vi "RDB Init New Message.vi"(7 "RDB Receive Reference.RDB Signals":dbl[](array[numeric]), 8 "error in (no error)":errorcluster, 10 "RDB Reference in":T4 {"RDB Send Reference"."RDB Data"."payload" format="%x"; "RDB Send Reference"."RDB Data"."timestamp" format="%<%.7X\n%x>T"; "RDB Send Reference"."RDB Data"."type" items=["FlexRay Data"=32, "FlexRay Null"=33, "FlexRay Symbol"=34, "Log Trigger"=225, "Start Trigger"=226]; "RDB Send Reference"."RDB Data"."cycle count" max=63 step=1; "RDB Receive Reference"."RDB Data"."payload" format="%x"; "RDB Receive Reference"."RDB Data"."timestamp" format="%<%.7X\n%x>T"; "RDB Receive Reference"."RDB Data"."type" items=["FlexRay Data"=32, "FlexRay Null"=33, "FlexRay Symbol"=34, "Log Trigger"=225, "Start Trigger"=226]; "RDB Receive Reference"."RDB Data"."cycle count" max=63 step=1}, 11 "Settings":T1={"UDP Receiver"=refnum, "UDP Sender"=refnum, "Valid Packet"=FALSE, "TCP"=refnum, "Network Settings"={"IP adress"="127.0.0.1", "RDB"={"Protocol"=enum."UDP", "Tx Port"=48270, "Rx Port"=10, "Buffer Size"=204800, "Timeout"=10}, "SCP"={"Protocol"=enum."TCP", "Tx Port"=48191, "Rx Port"=48191, "Buffer Size"=204800, "Timeout"=10}}, "vclient"=path ""}) -> (0 "error out":errorcluster, 2 "RDB Reference out":T4 {"RDB Send Reference"."RDB Data"."payload" format="%x"; "RDB Send Reference"."RDB Data"."timestamp" format="%<%.7X\n%x>T"; "RDB Send Reference"."RDB Data"."type" items=["FlexRay Data"=32, "FlexRay Null"=33, "FlexRay Symbol"=34, "Log Trigger"=225, "Start Trigger"=226]; "RDB Send Reference"."RDB Data"."cycle count" max=63 step=1; "RDB Receive Reference"."RDB Data"."payload" format="%x"; "RDB Receive Reference"."RDB Data"."timestamp" format="%<%.7X\n%x>T"; "RDB Receive Reference"."RDB Data"."type" items=["FlexRay Data"=32, "FlexRay Null"=33, "FlexRay Symbol"=34, "Log Trigger"=225, "Start Trigger"=226]; "RDB Receive Reference"."RDB Data"."cycle count" max=63 step=1}, 3 "Settings":T1={"UDP Receiver"=refnum, "UDP Sender"=refnum, "Valid Packet"=FALSE, "TCP"=refnum, "Network Settings"={"IP adress"="127.0.0.1", "RDB"={"Protocol"=enum."UDP", "Tx Port"=48270, "Rx Port"=10, "Buffer Size"=204800, "Timeout"=10}, "SCP"={"Protocol"=enum."TCP", "Tx Port"=48191, "Rx Port"=48191, "Buffer Size"=204800, "Timeout"=10}}, "vclient"=path ""})   [LabVIEW 2020, in "RDB.lvlib"]
uses:
  RDB.lvlib
  RDB References.ctl
  RDB Reference.ctl
  <vilib>/xnet/xnet.llb/XNET Frame FlexRay.ctl
  <vilib>/xnet/xnet.llb/XNET Frame Type FlexRay.ctl
  Engine/Type/Settings.ctl
  Shared/Network Settings.ctl
  Shared/Protocol.ctl
  <vilib>/xnet/xnet.llb/XNET Convert (Signal to Frame FlexRay).vi
  Shared/Vires VTD Shared.lvlib
  Engine/Vires VTD Engine.lvlib
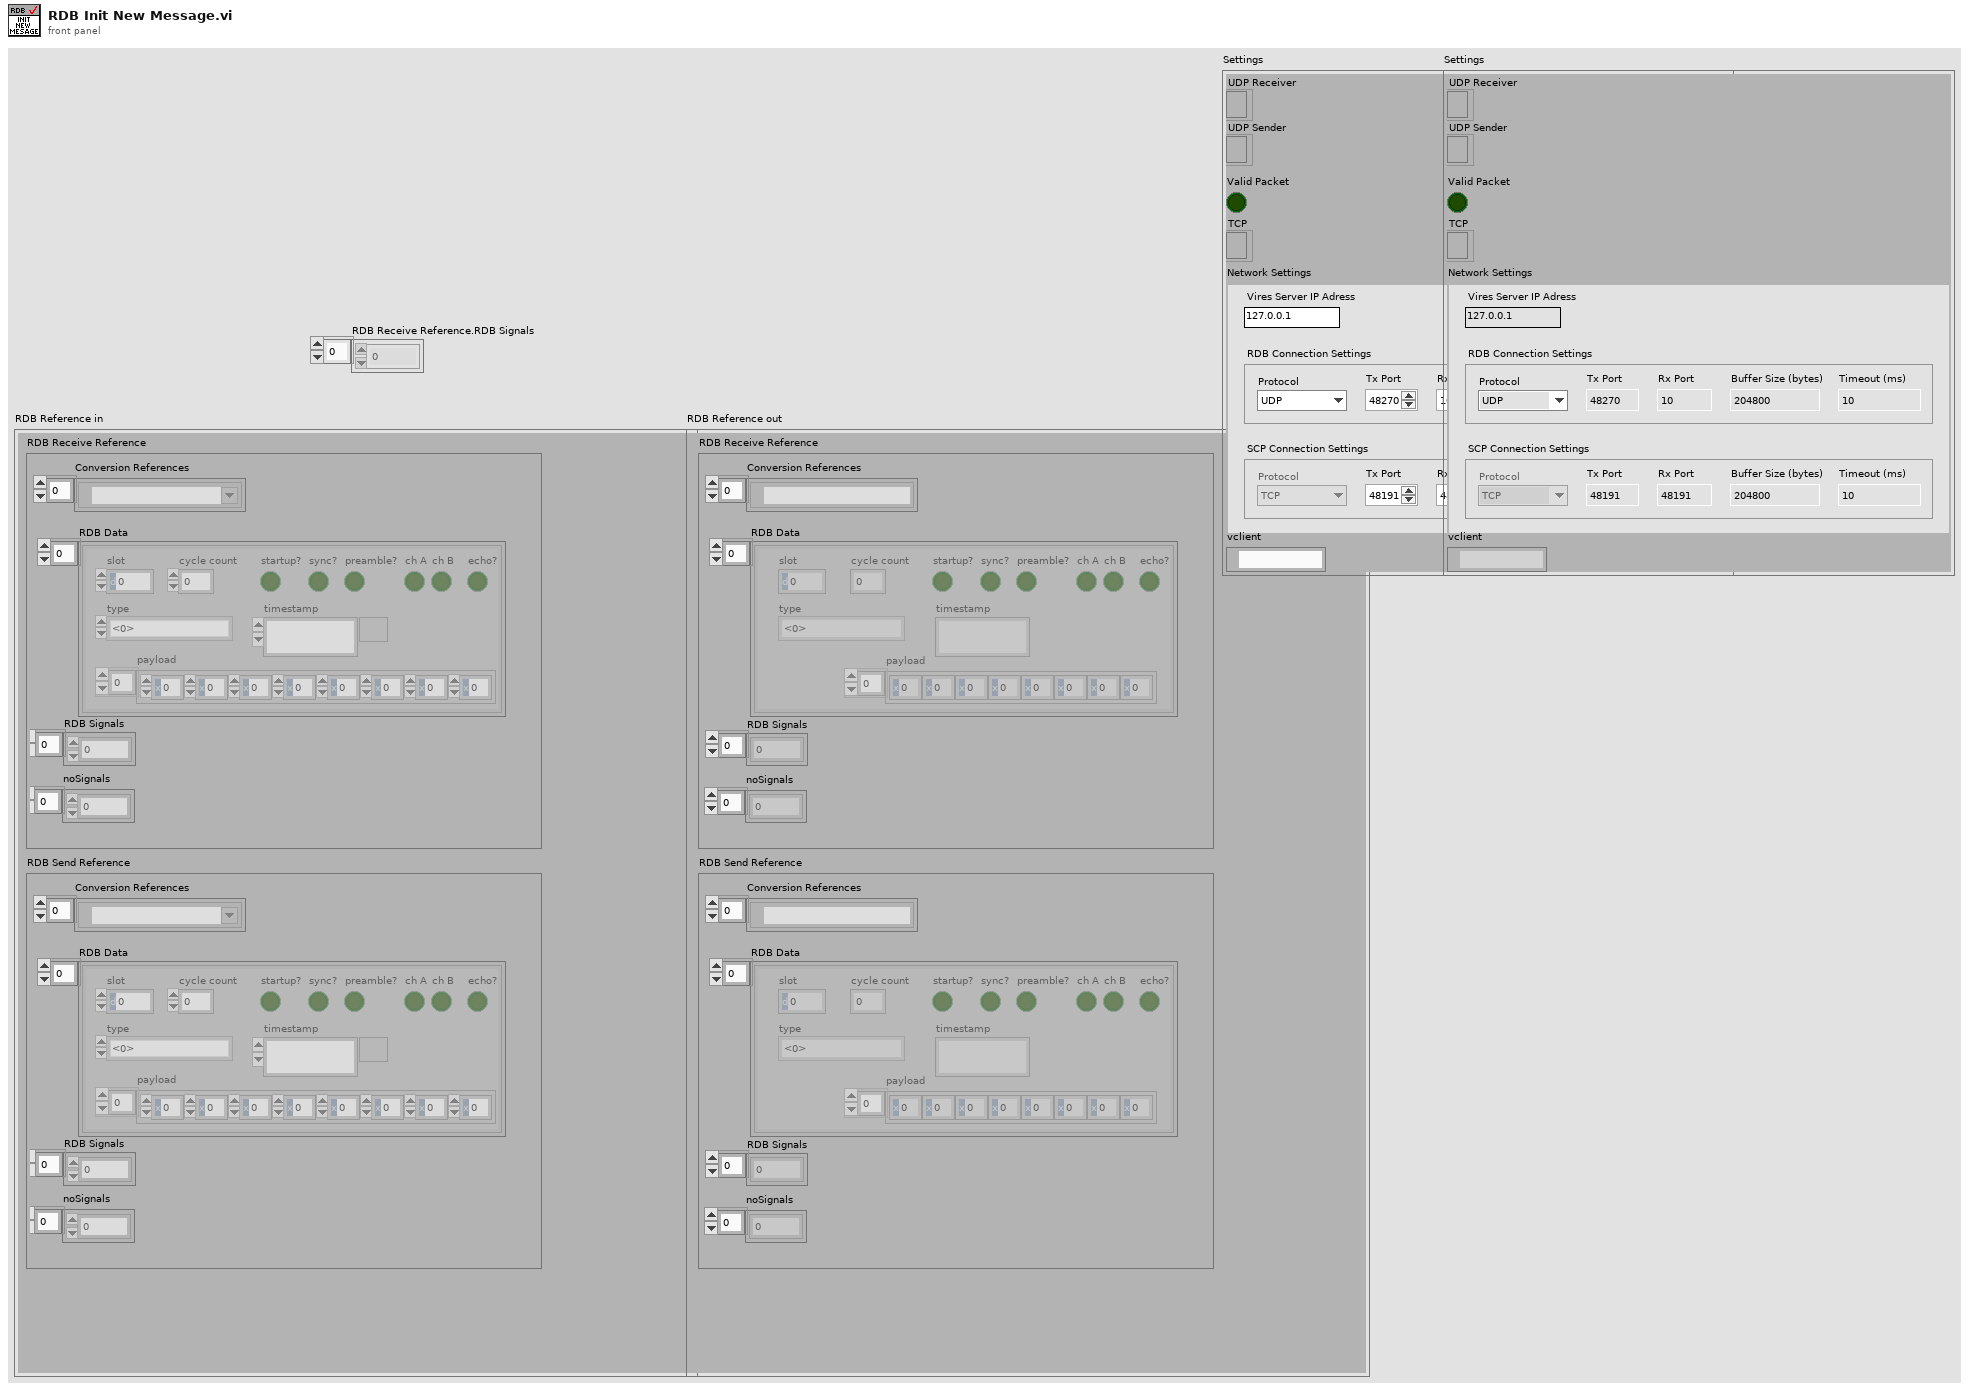
[diagram p1: front panel]
types:
  T1 = typedef "Vires VTD Engine.lvlib/Settings.ctl" = cluster{"UDP Receiver":refnum<k16>, "UDP Sender":refnum<k16>, "Valid Packet":bool, "TCP":refnum<k5>, "Network Settings":T2, "vclient":path}
  T2 = typedef "Vires VTD Shared.lvlib/Network Settings.ctl" = cluster{"IP adress":string, "RDB":cluster{"Protocol":T3, "Tx Port":u16, "Rx Port":u16, "Buffer Size":i32, "Timeout":u16}, "SCP":cluster{"Protocol":T3, "Tx Port":u16, "Rx Port":u16, "Buffer Size":i32, "Timeout":u16}}
  T3 = typedef "Vires VTD Shared.lvlib/Protocol.ctl" = enum16{"UDP", "TCP"}
  T4 = typedef "RDB.lvlib/RDB References.ctl" = cluster{"RDB Receive Reference":T5, "RDB Send Reference":T5}
  T5 = typedef "RDB.lvlib/RDB Reference.ctl" = cluster{"Conversion References":refnum<k21>[], "RDB Data":T6[], "RDB Signals":dbl[], "noSignals":i32[]}
  T6 = typedef "XNET Frame FlexRay.ctl" = cluster{"timestamp":timestamp, "payload":u8[], "slot":u16, "type":T7, "cycle count":u8, "startup?":bool, "sync?":bool, "preamble?":bool, "ch A":bool, "ch B":bool, "echo?":bool}
  T7 = typedef "XNET Frame Type FlexRay.ctl" = u8
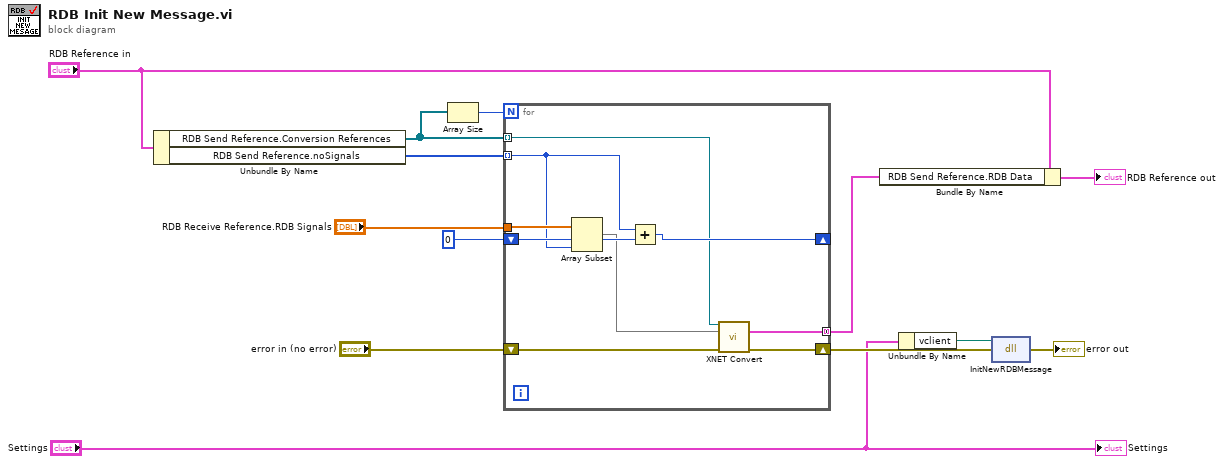
[diagram p0: block diagram]
diagram:
  n1 = Unbundle By Name("RDB Reference in") -> ("RDB Send Reference.Conversion References"=w4:refnum<k21>[], "RDB Send Reference.noSignals"=w3:i32[])
  n2 = Array Size(array=w4) -> (size(s)=w11:i32)
  n3 = for {
    N: w11 -> [_]
    shift-right: [w18] -> w6
    shift-left: "error in (no error)" -> [w15]
    tunnel: w4 -> [w16] mode=indexing
    tunnel: "RDB Receive Reference.RDB Signals" -> [w22]
    shift-right: [w20] -> _
    shift-left: 0 -> [w21]
    tunnel: [w17] -> w8 mode=concatenating
    tunnel: w3 -> [w14] mode=indexing
    n4 = Array Subset(array=w22, index=w21, length=w14) -> (w19:dbl[])
    n5 = Add(x=w14, y=w21) -> (x+y=w20:i32)
    n6 = call-poly <vilib>:"XNET Convert.vi"("session in"=w16, "signal data"=w19, "error in (no error)"=w15) -> ("frame data"=w17:T6[], "error out"=w18:errorcluster)  [unwired: 9 in, 2 out]
  }
  n7 = Bundle By Name(cluster="RDB Reference in", "RDB Send Reference.RDB Data"=w8) -> (→"RDB Reference out":T4)
  n8 = Unbundle By Name("Settings") -> ("vclient"=w1:path)
  n9 = dll-call lib="E:/Documents/Systems Engineering/Custom VeriStand Development/Vires VTD Custom Device/Vires VTD Custom Device/Vires VTD/Source/RDB/vclient.*" fn="InitNewRDBMessage"(path in=w1, error in=w6) -> (error out=→"error out":errorcluster)  [unwired: 2 in, 1 out]
  "Settings" <- "Settings"
